vi "find readout time.vi"(8 "error in (no error)":errorcluster, 11 "Simulated_CCD_Camera in":refnum<class "Simulated Camera.lvclass">) -> (0 "error out":errorcluster, 3 "Simulated_CCD_Camera out":refnum<class "Simulated Camera.lvclass">)   [LabVIEW 2018, in "Simulated Camera.lvclass"]
doc: "Find the readout time as a function of the operation mode of the CCD.\n\nThis value is used to determine the minimum exposure time allowed by ACS, that is the readout time plus 10 % of this value. This procedure is related to the functioning of the frame transfer mode of the CCD and it prevents the misuse of the exposure time."
uses:
  Simulated Camera.lvclass
  Simulated Camera.lvclass/Simulated Camera.ctl
  <vilib>/Utility/file.llb/Read Delimited Spreadsheet (DBL).vi
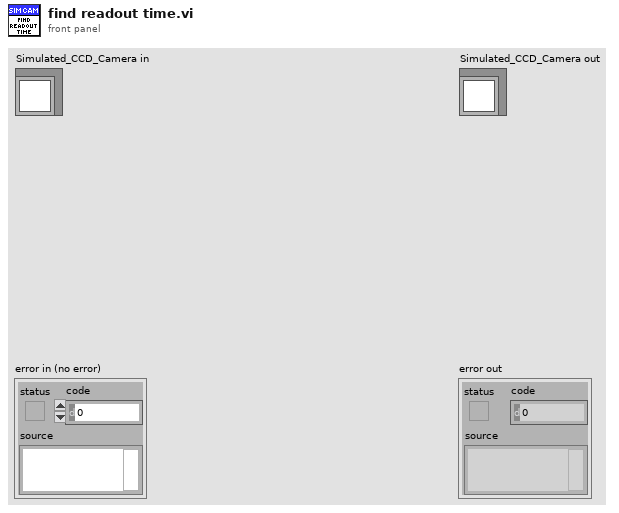
[diagram p1: front panel]
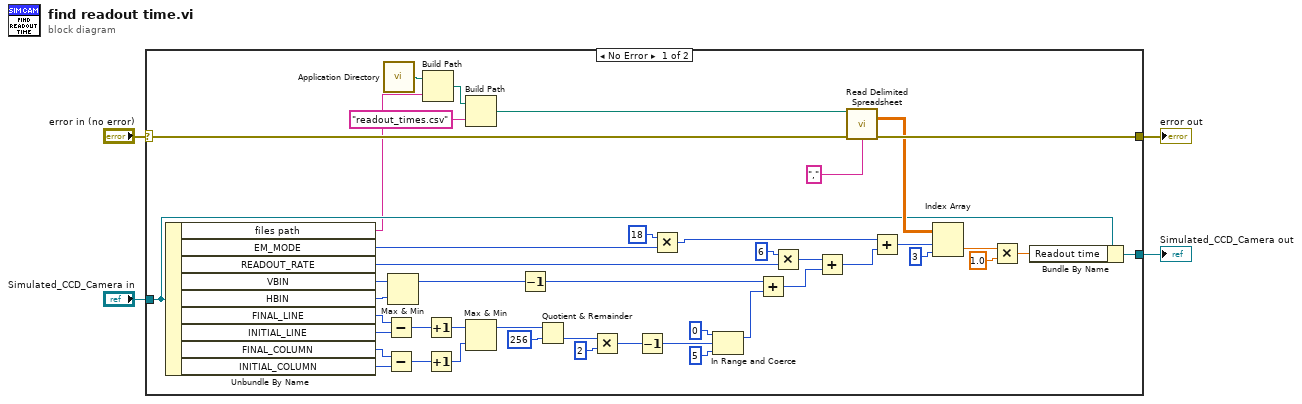
[diagram p0: block diagram]
diagram:
  n1 = case shown="No Error" "error in (no error)" {
    selector: "error in (no error)" -> [w49 w51]
    tunnel: [w48 w51] -> w3
    tunnel: [w10 w50] -> w1
    tunnel: "Simulated_CCD_Camera in" -> [w11 w50]
    frame No Error {
      n2 = Unbundle By Name(w11) -> ("files path"=w5:string, "EM_MODE"=w27:u16, "READOUT_RATE"=w31:u16, "VBIN"=w35:u16, "HBIN"=w34:u16, "FINAL_LINE"=w43:u16, "INITIAL_LINE"=w42:u16, "FINAL_COLUMN"=w41:u16, "INITIAL_COLUMN"=w40:u16)
      n3 = call <vilib>:"Application Directory.vi"() -> ("Application Directory"=w46:path)
      n4 = Subtract(x=w43, y=w42) -> (x-y=w45:u16)
      n5 = Subtract(x=w41, y=w40) -> (x-y=w44:u16)
      n6 = Max & Min(x=w35, y=w34) -> (max(x,y)=w33:u16)  [unwired: 1 out]
      n7 = Build Path(base path=w46, name or relative path=w5) -> (appended path=w8:path)
      n8 = Increment(x=w45) -> (x+1=w39:u16)
      n9 = Increment(x=w44) -> (x+1=w38:u16)
      n10 = Build Path(base path=w8, name or relative path="readout_times.csv") -> (appended path=w7:path)
      n11 = Max & Min(x=w39, y=w38) -> (max(x,y)=w36:u16)  [unwired: 1 out]
      n12 = Decrement(x=w33) -> (x-1=w32:u16)
      n13 = Quotient & Remainder(x=w36, y=u16 256) -> (floor(x/y)=w18:u16)  [unwired: 1 out]
      n14 = Multiply(x=w18, y=u16 2 ("x")) -> (x*y=w19:u16)
      n15 = Decrement(x=w19) -> (x-1=w17:u16)
      n16 = Multiply(x=u16 18, y=w27) -> (x*y=w24:u16)
      n17 = In Range and Coerce(upper limit=u16 0, x=w17, lower limit=u16 5 ("upper limit")) -> (coerced(x)=w14:u16)  [unwired: 1 out]
      n18 = Add(x=w32, y=w14) -> (x+y=w29:u16)
      n19 = Multiply(x=u16 6, y=w31) -> (x*y=w28:u16)
      n20 = Add(x=w28, y=w29) -> (x+y=w25:u16)
      n21 = call-poly <vilib>:"Read Delimited Spreadsheet.vi"("file path (dialog if empty)"=w7, "error in (no error)"=w49, "delimiter (\\t)"="," ("delimiter (\\t)")) -> ("all rows"=w23:dbl[][], "error out"=w48:errorcluster)  [unwired: 7 in, 4 out]
      n22 = Add(x=w24, y=w25) -> (x+y=w21:u16)
      n23 = Index Array(array=w23, index (row)=w21, index (col)=3 ("disabled index (col)")) -> (element=w13:dbl)
      n24 = Multiply(x=w13, y=1.0) -> (x*y=w9:dbl)
      n25 = Bundle By Name(cluster=w11, "Readout time"=w9) -> (w10:refnum<class "Simulated Camera.lvclass">)
    }
    frame Error {
    }
  }
  "error out" <- w3
  "Simulated_CCD_Camera out" <- w1
